vi "AH 2700 Continuous Measurement.vi"() -> ()   [LabVIEW 2019]
doc: "This example shows how to configure the bridge,initiate continuous capacitance measurement, read the results from the bridge, and parse the measurement results."
uses:
  Andeen-Hagerling 2700(400 firmware).lvlib
panel:
  out "Attentap":string
  out "Loss Greater Than":string
  in  "Total":i32 min=0 max=99999999
  in  "Interval":dbl min=0.0 max=99999999.0 step=0.1 format="%#_10f"
  out "Loss Chart":dbl(graph)
  out "Capacitance Chart":dbl(graph)
  out "Sample Switch":i32
  in  "stop":bool
  out "Frequency (Hz)":dbl
  out "Units Display":i32(ring)=1 items=["nanosiemens"=1, "dissipation factor"=2, "kilohms"=3, "gigohms"=4, "loss vector (jpF)"=5]
  out "Error Message":string
  out "Voltage (V)":dbl format="%#_6f"
  out "Loss":dbl
  out "Capacitance (pF)":dbl format="%#_10f"
  in  "Units":i32(ring)=1 items=["nanosiemens"=1, "dissipation factor"=2, "kilohms"=3, "gigohms"=4, "loss vector (jpF)"=5]
  in  "Bridge\nFrequency (Hz)":dbl(ring)=1000.0 items=["50"=50.0, "60"=60.0, "70"=70.0, "80"=80.0, "100"=100.0, "120"=120.0, "140"=140.0, "160"=160.0, "200"=200.0, "240"=240.0, "300"=300.0, "400"=400.0, "500"=500.0, "600"=600.0, "700"=700.0, "800"=800.0, "1000"=1000.0, "1200"=1200.0, "1400"=1400.0, "1600"=1600.0, "2000"=2000.0, "2400"=2400.0, "3000"=3000.0, "4000"=4000.0, "5000"=5000.0, "6000"=6000.0, "7000"=7000.0, "8000"=8000.0, "10000"=10000.0, "12000"=12000.0, "14000"=14000.0, "16000"=16000.0, "20000"=20000.0]
  in  "Maximum\nVoltage (V)":dbl=15.0 min=0.0003 max=15.0 step=1.0 format="%#.6f"
  in  "Average\nExponent":u16=4 max=15
  in  "VISA Resource":refnum<visa-resource-name>
  in  "Serial Configuration":T1={"Baud Rate"=9600, "Parity"=0, "Data Bits"=8, "Stop Bits"=10} {"Stop Bits" items=["1.0"=10, "1.5"=15, "2.0"=20]; "Data Bits" items=["7"=7, "8"=8]; "Parity" items=["None", "Odd", "Even", "Mark", "Space"]; "Baud Rate" items=["300"=300, "600"=600, "1200"=1200, "2400"=2400, "4800"=4800, "9600"=9600, "19200"=19200, "38400"=38400, "57600"=57600, "115200"=115200]}
  # "AH 2700A ULTRA-PRECISION 50Hz-20kHz CAPACITANCE BRIDGE"
  # "Continuous Measurement"
  # "Measurement Parameters"
  # "Continuous Parameters"
  # "Measurement Results"
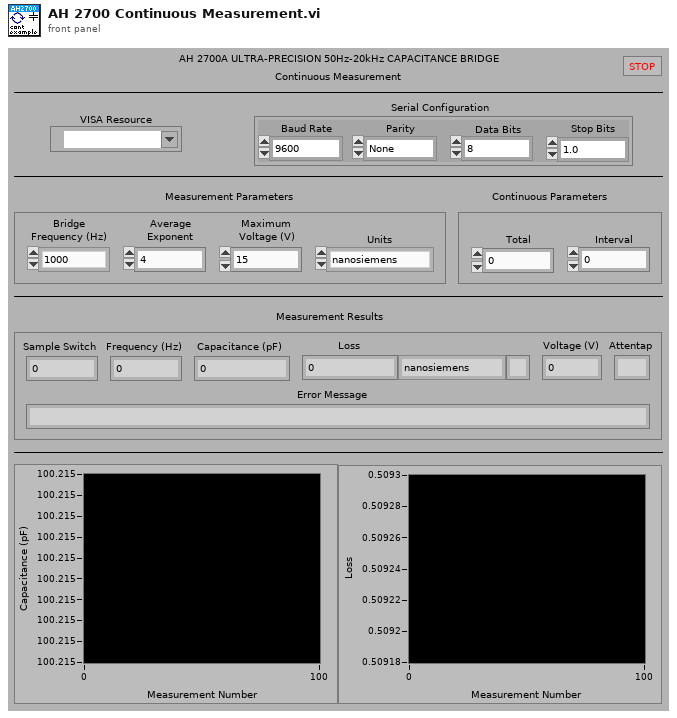
[diagram p1: front panel]
types:
  T1 = cluster{"Baud Rate":u32, "Parity":u16, "Data Bits":u16, "Stop Bits":u16}
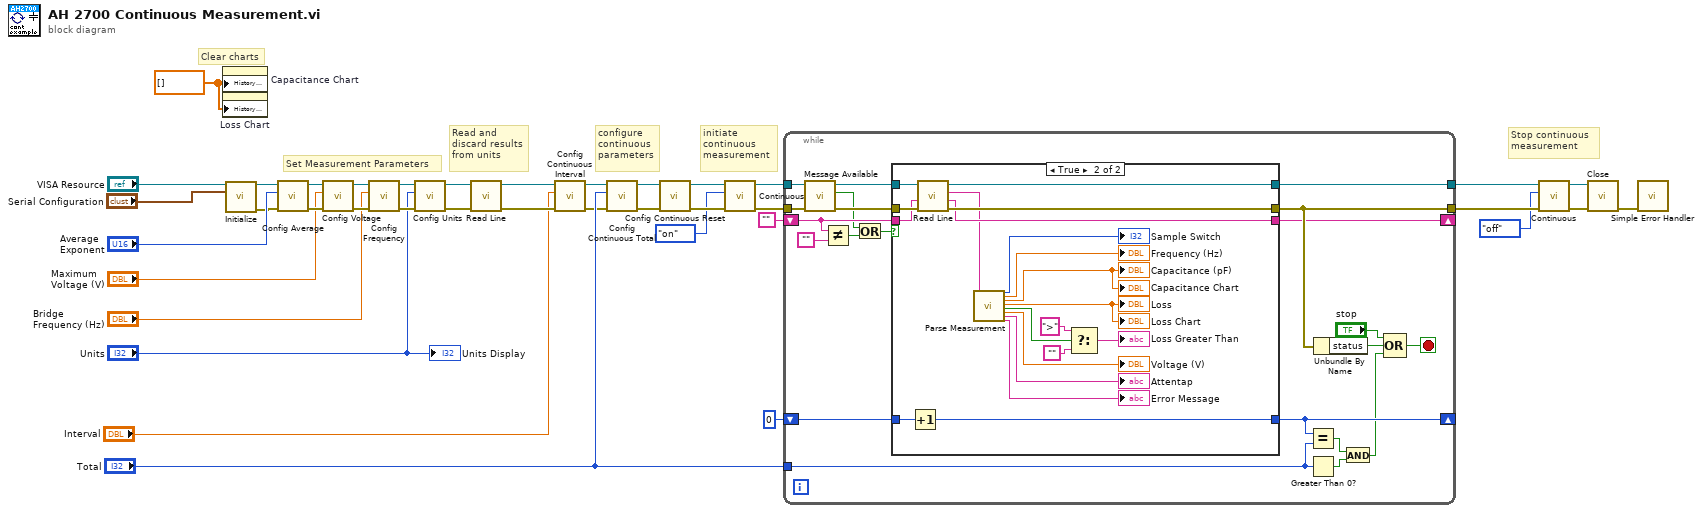
[diagram p0: block diagram]
diagram:
  w19 = dbl[] [] ("History Data")
  # "configure\ncontinuous\nparameters"
  # "Clear charts"
  # "Stop continuous\nmeasurement"
  # "initiate\ncontinuous\nmeasurement"
  # "Set Measurement Parameters"
  # "Read and\ndiscard results\nfrom units"
  n1 = property on="Capacitance Chart" class="WFChart (strict)"("History Data"=w19) -> ()  [unwired: 2 in, 2 out]
  n2 = property on="Loss Chart" class="WFChart (strict)"("History Data"=w19) -> ()  [unwired: 2 in, 2 out]
  n3 = call "Initialize.vi"("VISA resource name"="VISA Resource", "Serial Configuration"="Serial Configuration") -> ("VISA resource name out"=w4:refnum<visa-resource-name>, "error out"=w3:errorcluster)  [unwired: 12 in]
  n4 = call "Config Average.vi"("error in"=w3, "Average Exponent (4)"="Average\nExponent", "VISA resource name"=w4) -> ("error out"=w35:errorcluster, "VISA resource name out"=w38:refnum<visa-resource-name>)  [unwired: 7 in]
  n5 = call "Config Voltage.vi"("error in"=w35, "Voltage (15 V)"="Maximum\nVoltage (V)", "VISA resource name"=w38) -> ("error out"=w34:errorcluster, "VISA resource name out"=w37:refnum<visa-resource-name>)  [unwired: 7 in]
  n6 = call "Config Frequency.vi"("error in"=w34, "Frequency (1000 Hz)"="Bridge\nFrequency (Hz)", "VISA resource name"=w37) -> ("error out"=w33:errorcluster, "VISA resource name out"=w36:refnum<visa-resource-name>)  [unwired: 7 in]
  n7 = call "Config Units.vi"("error in"=w33, "Units (nS)"="Units", "VISA resource name"=w36) -> ("error out"=w28:errorcluster, "VISA resource name out"=w29:refnum<visa-resource-name>)  [unwired: 7 in]
  n8 = call "Read Line.vi"("error in"=w28, "VISA resource name"=w29) -> ("error out"=w10:errorcluster, "VISA resource name out"=w11:refnum<visa-resource-name>)  [unwired: 6 in, 2 out]
  n9 = call "Config Continuous Interval.vi"("error in"=w10, "Interval (0)"="Interval", "VISA resource name"=w11) -> ("error out"=w8:errorcluster, "VISA resource name out"=w9:refnum<visa-resource-name>)  [unwired: 7 in]
  n10 = call "Config Continuous Total.vi"("error in"=w8, "Total (0)"="Total", "VISA resource name"=w9) -> ("error out"=w14:errorcluster, "VISA resource name out"=w15:refnum<visa-resource-name>)  [unwired: 7 in]
  n11 = call "Config Continuous Reset.vi"("error in"=w14, "VISA resource name"=w15) -> ("error out"=w13:errorcluster, "VISA resource name out"=w12:refnum<visa-resource-name>)  [unwired: 6 in]
  n12 = call "Continuous.vi"("error in"=w13, "Scan Measurement (on)"=enum16{"off", "on"}."on", "VISA resource name"=w12) -> ("error out"=w25:errorcluster, "VISA resource name out"=w26:refnum<visa-resource-name>)  [unwired: 7 in]
  n13 = while {
    tunnel: [w59] -> w21
    tunnel: [w58] -> w23
    tunnel: w26 -> [w56]
    tunnel: w25 -> [w54]
    shift-right: [w57] -> _
    shift-left: "" -> [w42]
    shift-right: [w51] -> _
    shift-left: 0 -> [w52]
    tunnel: "Total" -> [w47]
    stop <- w49 stop-if-true
    n14 = call "Message Available.vi"("error in"=w54, "VISA resource name"=w56) -> ("error out"=w53:errorcluster, "message available"=w40:bool, "VISA resource name out"=w55:refnum<visa-resource-name>)  [unwired: 7 in]
    n15 = Not Equal?(x=w42, y="") -> (x != y?=w41:bool)
    n16 = Or(x=w40, y=w41) -> (x .or. y?=w39:bool)
    n17 = case shown="True" w39 {
      tunnel: [w63 w83] -> w59
      tunnel: w55 -> [w63 w82]
      tunnel: w53 -> [w62 w81]
      tunnel: [w62 w80] -> w58
      tunnel: [w61 w76] -> w57
      tunnel: w42 -> [w61 w77]
      tunnel: w52 -> [w60 w79]
      tunnel: [w60 w78] -> w51
      frame False {
      }
      frame True {
        n18 = Increment(x=w79) -> (x+1=w78:i32)
        n19 = call "Read Line.vi"("error in"=w81, "Previous"=w77, "VISA resource name"=w82) -> ("error out"=w80:errorcluster, "Remaining"=w76:string, "Message"=w75:string, "VISA resource name out"=w83:refnum<visa-resource-name>)  [unwired: 5 in]
        n20 = call "Parse Measurement.vi"("Measurement Line"=w75) -> ("Sample"=→"Sample Switch":i32, "Frequency"=→"Frequency (Hz)":dbl, "Capacitance"=→"Capacitance (pF)" →"Capacitance Chart":dbl, "Loss"=→"Loss" →"Loss Chart":dbl, "Loss Greater Than"=w70:bool, "Voltage"=→"Voltage (V)":dbl, "Attentap"=→"Attentap":string, "Error Message"=→"Error Message":string)  [unwired: 17 in, 2 out]
        n21 = Select(t=">", s=w70, f="") -> (s? t:f=→"Loss Greater Than":string)
      }
    }
    n22 = Equal?(x=w51, y=w47) -> (x = y?=w46:bool)
    n23 = Greater Than 0?(x=w47) -> (x > 0?=w45:bool)
    n24 = Unbundle By Name(w58) -> ("status"=w50:bool)
    n25 = And(x=w46, y=w45) -> (x .and. y?=w44:bool)
    n26 = Compound Arithmetic op=OR("stop", w50, w44) -> (w49:bool)
  }
  n27 = call "Continuous.vi"("error in"=w23, "Scan Measurement (on)"=enum16{"off", "on"}."off", "VISA resource name"=w21) -> ("error out"=w24:errorcluster, "VISA resource name out"=w22:refnum<visa-resource-name>)  [unwired: 7 in]
  n28 = call "Close.vi"("error in (no error)"=w24, "VISA resource name"=w22) -> ("error out"=w20:errorcluster)  [unwired: 9 in]
  n29 = call <vilib>:"Simple Error Handler.vi"("error in (no error)"=w20) -> ()  [unwired: 4 in, 5 out]
  "Units Display" <- "Units"
